vi "CANTest.vi"() -> ()   [LabVIEW 2009]
uses:
  SubVIs/CAN Jaguar Control Mode.ctl
  SubVIs/CAN Jaguar Position Reference.ctl
  <vilib>/Platform/TimedLoop/XDataNode/XDataNode.xnode
  <vilib>/Platform/TimedLoop/XDataNode/loadlvalarms.vi
  <vilib>/Platform/TimedLoop/XDataNode/timing_clust.ctl
  <vilib>/Platform/TimedLoop/XDataNode/nitl_modes.ctl
  <vilib>/Platform/TimedLoop/XDataNode/wakeup.ctl
  Serial.lvlib
  <vilib>/Platform/TimedLoop/XDataNode/XDNodeRunTimeDep.lvlib
  CAN.lvlib
panel:
  out "D 2":dbl
  out "I 2":dbl
  out "P 2":dbl
  out "Output Set Point 2":dbl
  in  "Maximum Output Voltage":dbl
  in  "D":dbl
  in  "I":dbl
  in  "P":dbl
  in  "Device Number":u8
  out "error out 2":errorcluster
  out "error out":errorcluster
  in  "stop":bool
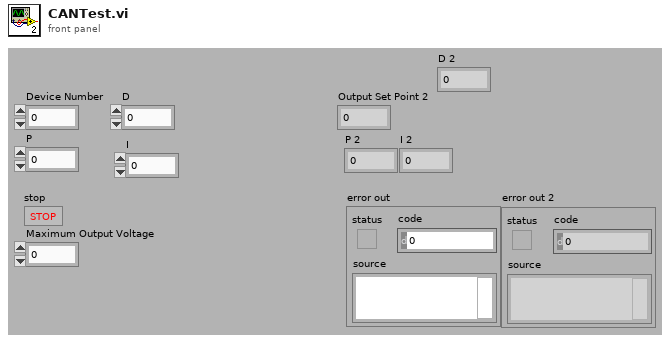
[diagram p1: front panel]
types:
  T1 = typedef "CAN.lvlib/CAN Jaguar Position Reference.ctl" = enum16{"Encoder", "Potentiometer"}
  T2 = typedef "CAN.lvlib/CAN Jaguar Control Mode.ctl" = enum16{"Percent VBus", "Speed", "Position", "Current"}
  T3 = typedef "XDNodeRunTimeDep.lvlib/timing_clust.ctl" = cluster{"Expected End [f-1]":u64, "Actual End [f-1]":u64, "Finished Late? [f-1]":bool, "Expected End [i-1]":u64, "Actual End [i-1]":u64, "Finished Late? [i-1]":bool, "Expected Start [i]":u64, "Actual Start [i]":u64, "Expected Start [f]":u64, "Actual Start [f]":u64, "Source Name":string, "Structure Name":string, "Period":i64, "Deadline":i64, "Offset":i64, "Start":i64, "Priority":i32, "Timeout":i32, "Mode":T4, "Wakeup Reason":T5, "Error":errorcluster, "Source Type":string, "Secondary Source Type":string, "Global End Time":u64, "Global Start Time":u64, "Frame Duration":u64, "Iteration Duration":u64, "Assigned CPU":i32, "I/O Scan Engine Mode":u32}
  T4 = typedef "XDNodeRunTimeDep.lvlib/nitl_modes.ctl" = enum32{"No Change", "Process missed periods, maintain original phase", "Discard missed periods, maintain original phase", "Process missed periods, ignore original phase", "Discard missed periods, ignore original phase"}
  T5 = typedef "XDNodeRunTimeDep.lvlib/wakeup.ctl" = enum32{"Normal", "Aborted", "Asynchronous wakeup", "Timing source error", "Timed loop error", "Timeout"}
  T6 = typedef "CAN.lvlib/CAN Jaguar Ref.ctl" = cluster{"Device Number":u8, "Control Mode":T2, "Inverted":bool, "Semaphore":T7, "Max Vout":dbl, "DevStatus":errorcluster}
  T7 = typedef "Semaphore RefNum" = refnum<k1>
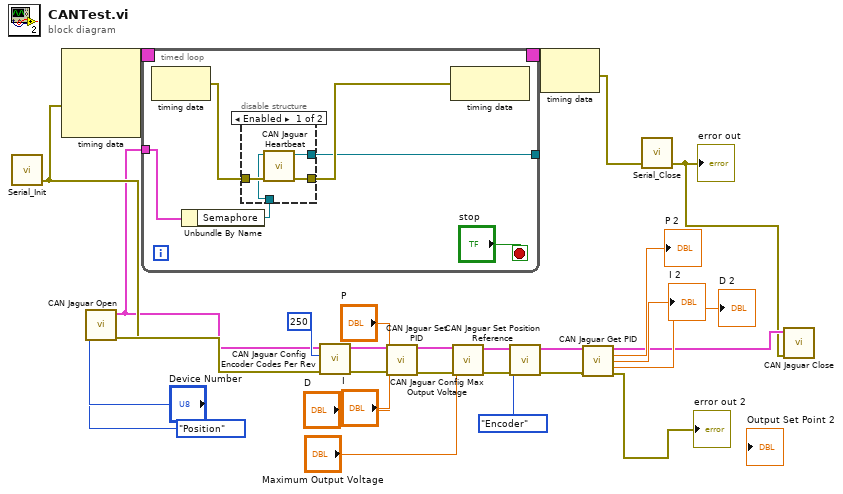
[diagram p0: block diagram]
diagram:
  n1 = call "Serial_Init.vi"() -> ("error out"=w5:errorcluster)  [unwired: 4 in, 1 out]
  n2 = node-c288(w5) -> (w28:T3)  [unwired: 3 in]
  n3 = call "CAN Jaguar Open.vi"("error in (no error)"=w5, "Control Mode"=CAN_Jaguar_Control_Mode."Position", "Device Number"="Device Number") -> ("error out"=w23:errorcluster, "CAN Jaguar Ref Out"=w4:T6)  [unwired: 7 in]
  n4 = timed-loop {
    timing: w28 -> [_]
    timing-out: [_] -> w27
    tunnel: w4 -> [w30]
    tunnel: [w31] -> _
    stop <- "stop" stop-if-true
    n5 = node-c288() -> (w34:errorcluster)  [unwired: 1 in]
    n6 = Unbundle By Name(w30) -> ("Semaphore"=w29:T7)
    n7 = disable-structure shown="Enabled" {
      disable-tunnel: w34 -> [w38 _]
      disable-tunnel: [w37 _] -> w33
      disable-tunnel: [w36 _] -> w31
      disable-tunnel: w29 -> [w35 _]
      frame #0 {
        n8 = call "CAN Jaguar Heartbeat.vi"("error in (no error)"=w38, "semaphore"=w35) -> ("error out"=w37:errorcluster, "semaphore out"=w36:T7)  [unwired: 8 in]
      }
      frame #1 {
      }
    }
    n9 = node-c288(w33) -> ()  [unwired: 1 out]
  }
  n10 = call "CAN Jaguar Config Encoder Codes Per Rev.vi"("error in (no error)"=w23, "Encoder Codes Per Rev"=u16 250, "CAN Jaguar Ref"=w4) -> ("error out"=w20:errorcluster, "CAN Jaguar Ref Out"=w21:T6)  [unwired: 7 in]
  n11 = call "CAN Jaguar Set PID.vi"("CAN Jaguar Ref"=w21, "P"="P", "I"="I", "D"="D", "error in (no error)"=w20) -> ("CAN Jaguar Ref Out"=w16:T6, "error out"=w15:errorcluster)  [unwired: 9 in]
  n12 = call "CAN Jaguar Config Max Output Voltage.vi"("error in (no error)"=w15, "Maximum Output Voltage"="Maximum Output Voltage", "CAN Jaguar Ref"=w16) -> ("error out"=w12:errorcluster, "CAN Jaguar Ref Out"=w13:T6)  [unwired: 7 in]
  n13 = call "CAN Jaguar Set Position Reference.vi"("error in (no error)"=w12, "Position Reference"=CAN_Jaguar_Position_Reference."Encoder", "CAN Jaguar Ref"=w13) -> ("error out"=w9:errorcluster, "CAN Jaguar Ref Out"=w10:T6)  [unwired: 7 in]
  n14 = node-c288(w27) -> (w26:errorcluster)
  n15 = call "CAN Jaguar Get PID.vi"("CAN Jaguar Ref"=w10, "error in (no error)"=w9) -> ("CAN Jaguar Ref Out"=w2:T6, "P"=→"P 2":dbl, "I"=→"I 2":dbl, "D"=→"D 2":dbl, "error out"=→"error out 2":errorcluster)  [unwired: 9 in]
  n16 = call "Serial_Close.vi"("error in (no error)"=w26) -> ("error out"=w1:errorcluster)  [unwired: 4 in]
  "error out" <- w1
  n17 = call "CAN Jaguar Close.vi"("error in (no error)"=w1, "CAN Jaguar Ref"=w2) -> ()  [unwired: 9 in, 1 out]
